vi "Write Errors.vi"(8 "error in (no error)":errorcluster, 11 "Data Value Reference in":refnum<data-value>) -> (0 "error out":errorcluster)   [LabVIEW 2015, in "Modbus Master Engine.lvlib"]
uses:
  Modbus Master Engine.lvlib
  <vilib>/addons/Inline Async API/_Data Access Engine/Access Type Classes/Write/Write.lvclass
  <vilib>/addons/Inline Async API/_Data Access Engine/Access Type Classes/Write/Write.lvclass/Write.ctl
  <vilib>/addons/Inline Async API/_Data Access Engine/Data Access Engine/Methods/Write.Data.vi
  <vilib>/addons/Inline Async API/_Data Access Engine/Access Type Classes/Write/Write.ProcessData.vi
  <vilib>/addons/Inline Async API/_Data Access Engine/Data Access Engine/Data Access Engine.lvclass
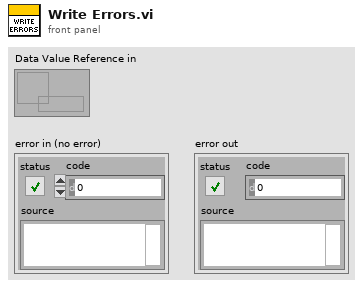
[diagram p1: front panel]
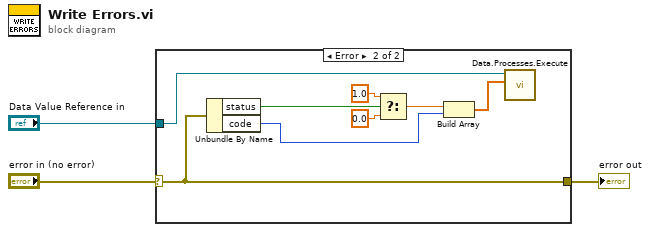
[diagram p0: block diagram]
diagram:
  n1 = case shown="Error" "error in (no error)" {
    selector: "error in (no error)" -> [w4 w6]
    tunnel: "Data Value Reference in" -> [_ w12]
    tunnel: [w4 w6] -> w1
    frame No Error {
    }
    frame Error {
      n2 = Unbundle By Name(w6) -> ("status"=w5:bool, "code"=w8:i32)
      n3 = Select(t=1.0, s=w5, f=0.0) -> (s? t:f=w9:dbl)
      n4 = Build Array(w9, w8) -> (w7:dbl[])
      n5 = call-poly <vilib>:"Data.Processes.Execute.vi"("Values"=w7, "Ref"=w12) -> ()  [unwired: 9 in, 1 out]
    }
  }
  "error out" <- w1
